vi "fgt get pressure Range.vi"(8 "error in (no error)":errorcluster, 11 "pressureIndex":u32) -> (0 "error out":errorcluster, 2 "Pmax out":sgl, 3 "Pmin out":sgl)   [LabVIEW 2020, in "fgt_SDK.lvlib"]
doc: "Get pressure controller minimum and maximum range. Returned values takes into account set unit, default value is 'mbar'."
uses:
  fgt_SDK.lvlib
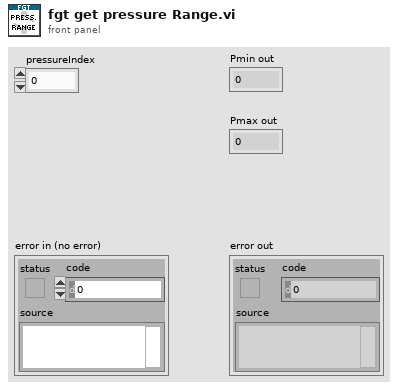
[diagram p1: front panel]
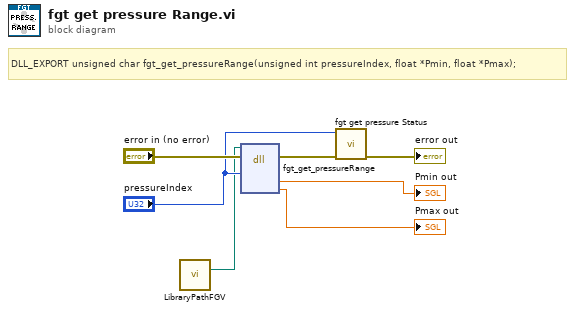
[diagram p0: block diagram]
diagram:
  # "DLL_EXPORT unsigned char fgt_get_pressureRange(unsigned int pressureIndex, float *Pmin, float *Pmax);"
  n1 = call "LibraryPathFGV.vi"() -> ("Path Out"=w1:path)  [unwired: 14 in, 1 out]
  n2 = dll-call lib="C:/Workspace/fgt-SDK/LabVIEW/dlls/fgt_SDK_*.*" fn="fgt_get_pressureRange"(path in=w1, error in="error in (no error)", "pressureIndex"="pressureIndex") -> (error out=w4:errorcluster, "Pmin"=→"Pmin out":sgl, "Pmax"=→"Pmax out":sgl)  [unwired: 5 in, 1 out]
  n3 = call "fgt get pressure Status.vi"("error in (no error)"=w4, "pressureIndex"="pressureIndex") -> ("error out"=→"error out":errorcluster)  [unwired: 9 in]
